vi "SetTilesQueue.vi"(8 "error in (no error)":errorcluster, 9 "Position":T1={"x"=-1.0, "y"=-1.0}, 10 "TileCodes":u16[][](array[numeric]), 11 "Game in":refnum<class "Game.lvclass">) -> (0 "error out":errorcluster, 3 "Game out":refnum<class "Game.lvclass">)   [LabVIEW 2019, in "RT_Game.lvlib" / "Game.lvclass"]
uses:
  Game.lvclass
  Coordinate.ctl
  Game.lvclass/Game.ctl
  Engine/Engine.lvclass
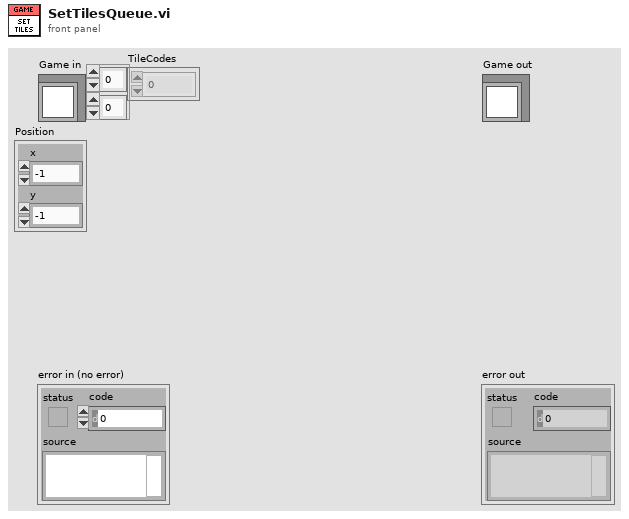
[diagram p1: front panel]
types:
  T1 = typedef "RT_Game.lvlib/Game.lvclass/Coordinate.ctl" = cluster{"x":dbl, "y":dbl}
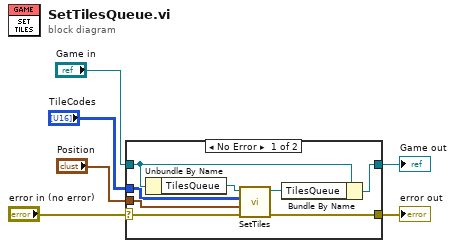
[diagram p0: block diagram]
diagram:
  n1 = case shown="No Error" "error in (no error)" {
    selector: "error in (no error)" -> [w14 w16]
    tunnel: [w13 w16] -> w5
    tunnel: [w10 w15] -> w3
    tunnel: "Game in" -> [w12 w15]
    tunnel: "Position" -> [w8 _]
    tunnel: "TileCodes" -> [w7 _]
    frame No Error {
      n2 = Unbundle By Name(w12) -> ("TilesQueue"=w11:refnum<queue>)
      n3 = call "SetTiles.vi"("error in (no error)"=w14, "Position"=w8, "TileCodes"=w7, "TilesQueue"=w11) -> ("error out"=w13:errorcluster, "TilesQueue out"=w9:refnum<queue>)  [unwired: 6 in]
      n4 = Bundle By Name(cluster=w12, "TilesQueue"=w9) -> (w10:refnum<class "Game.lvclass">)
    }
    frame Error {
    }
  }
  "error out" <- w5
  "Game out" <- w3
